vi "Write Notes.vi"(8 "error in (no error)":errorcluster, 10 "Notes":string, 11 "Step in":refnum<class "Step.lvclass">) -> (0 "error out":errorcluster, 3 "Step out":refnum<class "Step.lvclass">)   [LabVIEW 2020, in "MacroAssert.lvlib" / "Step.lvclass"]
uses:
  Step.lvclass
  Step.lvclass/Step.ctl
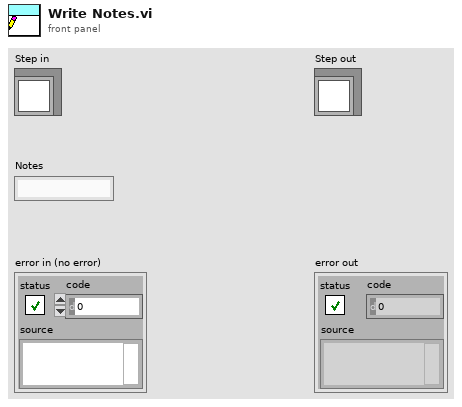
[diagram p1: front panel]
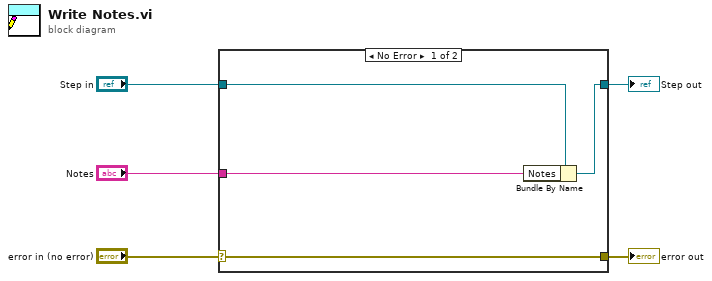
[diagram p0: block diagram]
diagram:
  n1 = case shown="No Error" "error in (no error)" {
    selector: "error in (no error)" -> [w9 w10]
    tunnel: [w9 w10] -> w4
    tunnel: [w7 w11] -> w2
    tunnel: "Step in" -> [w8 w11]
    tunnel: "Notes" -> [w6 _]
    frame No Error {
      n2 = Bundle By Name(cluster=w8, "Notes"=w6) -> (w7:refnum<class "Step.lvclass">)
    }
    frame Error {
    }
  }
  "error out" <- w4
  "Step out" <- w2
